vi "Write User Trigger Settings Reference.vi"(8 "error in (no error)":errorcluster, 10 "User_Trigger_Settings_Ref":refnum<vi>, 11 "AnalogInput in":refnum<class "AnalogInput.lvclass">) -> (0 "error out":errorcluster, 3 "AnalogInput out":refnum<class "AnalogInput.lvclass">)   [LabVIEW 2019, in "AnalogInput.lvlib" / "AnalogInput.lvclass"]
uses:
  Library/AnalogInput.lvclass
  Library/AnalogInput.lvclass/AnalogInput.ctl
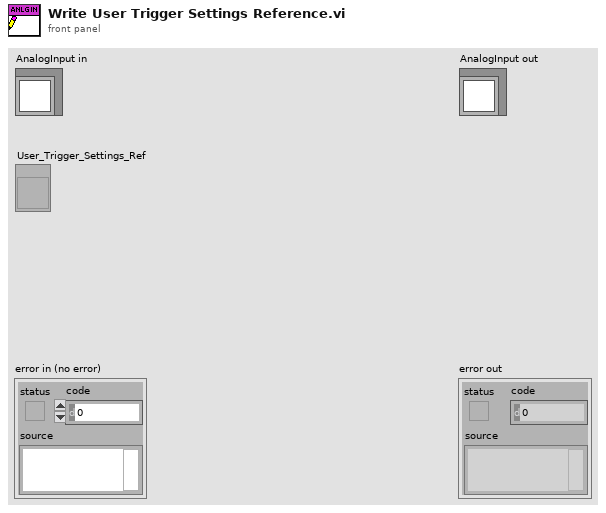
[diagram p1: front panel]
types:
  T1 = typedef "AnalogInput.lvlib/AnalogInput.lvclass/User Trigger Settings.ctl" = cluster{"Timeout":dbl, "Level":dbl, "Slope":T2, "samples per channel":i32, "Sample Rate (10k)":dbl, "pretrigger samples":u32}
  T2 = typedef "AnalogInput.lvlib/AnalogInput.lvclass/Trigger_Slope.ctl" = enum16{"Rising", "Falling"}
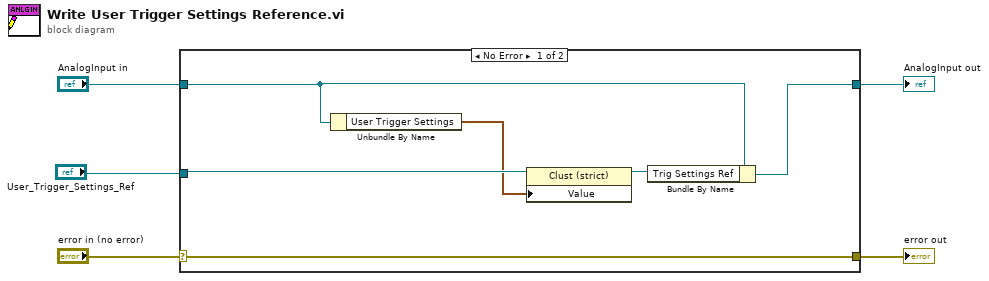
[diagram p0: block diagram]
diagram:
  n1 = case shown="No Error" "error in (no error)" {
    selector: "error in (no error)" -> [w11 w12]
    tunnel: [w11 w12] -> w4
    tunnel: [w10 w13] -> w2
    tunnel: "AnalogInput in" -> [w9 w13]
    tunnel: "User_Trigger_Settings_Ref" -> [w8 _]
    frame No Error {
      n2 = Unbundle By Name(w9) -> ("User Trigger Settings"=w6:T1)
      n3 = property class="Clust (strict)"(reference=w8, "Value"=w6) -> (reference out=w7:refnum<vi>)  [unwired: 1 in, 1 out]
      n4 = Bundle By Name(cluster=w9, "Trig Settings Ref"=w7) -> (w10:refnum<class "AnalogInput.lvclass">)
    }
    frame Error {
    }
  }
  "error out" <- w4
  "AnalogInput out" <- w2
